vi "DriveSetSpeedDemand.vi"(9 "ASpeedDemand (d/s)":dbl, 10 "YSpeedDemand (ft/s)":dbl, 11 "XSpeedDemand (ft/s)":dbl) -> ()   [LabVIEW 2020]
doc: "set speed demand variable for drive (called in human)"
uses:
  DriveGlobal.vi
  <vilib>/Rock Robotics/WPI/ThirdParty/JAS_Junk/TrajLib/Trajectory_Library.lvlib
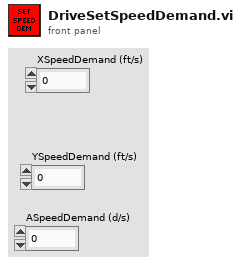
[diagram p1: front panel]
types:
  T1 = typedef "Trajectory_Library.lvlib/CHASSIS_SPEEDS.ctl" = cluster{"vX":dbl, "vY":dbl, "vOmega":dbl}
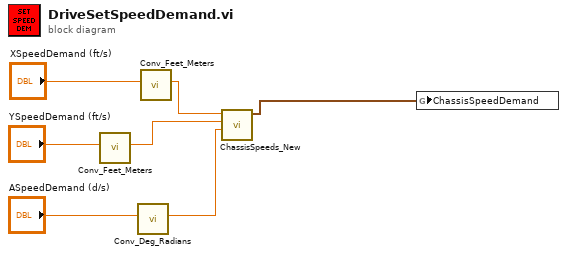
[diagram p0: block diagram]
diagram:
  n1 = call <vilib>:"Conv_Feet_Meters.vi"("Feet"="YSpeedDemand (ft/s)") -> ("Meters"=w3:dbl)  [unwired: 10 in]
  n2 = call <vilib>:"Conv_Deg_Radians.vi"("Degress"="ASpeedDemand (d/s)") -> ("Radians"=w5:dbl)  [unwired: 10 in]
  n3 = call <vilib>:"Conv_Feet_Meters.vi"("Feet"="XSpeedDemand (ft/s)") -> ("Meters"=w1:dbl)  [unwired: 10 in]
  n4 = call <vilib>:"ChassisSpeeds_New.vi"("vAngular"=w5, "vY"=w3, "vX"=w1) -> ("CHASSIS"=w7:T1)  [unwired: 8 in]
  n5 = global write "DriveGlobal.vi" "ChassisSpeedDemand"(w7) -> ()
